vi "Main.vi"(8 "error in (no error)":errorcluster, 11 "Data":T1) -> (0 "error out":errorcluster)   [LabVIEW 2020, in "Queue State Machine Lib.lvlib"]
doc: "Use this template to build a simple state machine design pattern. Each state executes code and determines which state to transition to."
uses:
  Queue State Machine Lib.lvlib
  controls/Data.ctl
  State Machine Data Class/State Machine Data Class.lvclass
  controls/State.ctl
  <vilib>/Delacor/Delacor QMH/Libraries/Message Queue_class/Delacor_lib_QMH_Message Queue.lvclass/Delacor_lib_QMH_Message Queue.ctl
  <vilib>/Delacor/Delacor QMH/Libraries/Message Queue_class/Delacor_lib_QMH_Enqueue Message (Single).vi
  <vilib>/Delacor/Delacor QMH/Libraries/Message Queue_class/Delacor_lib_QMH_Message Queue.lvclass
panel:
  in  "Multiple Consumer?":bool
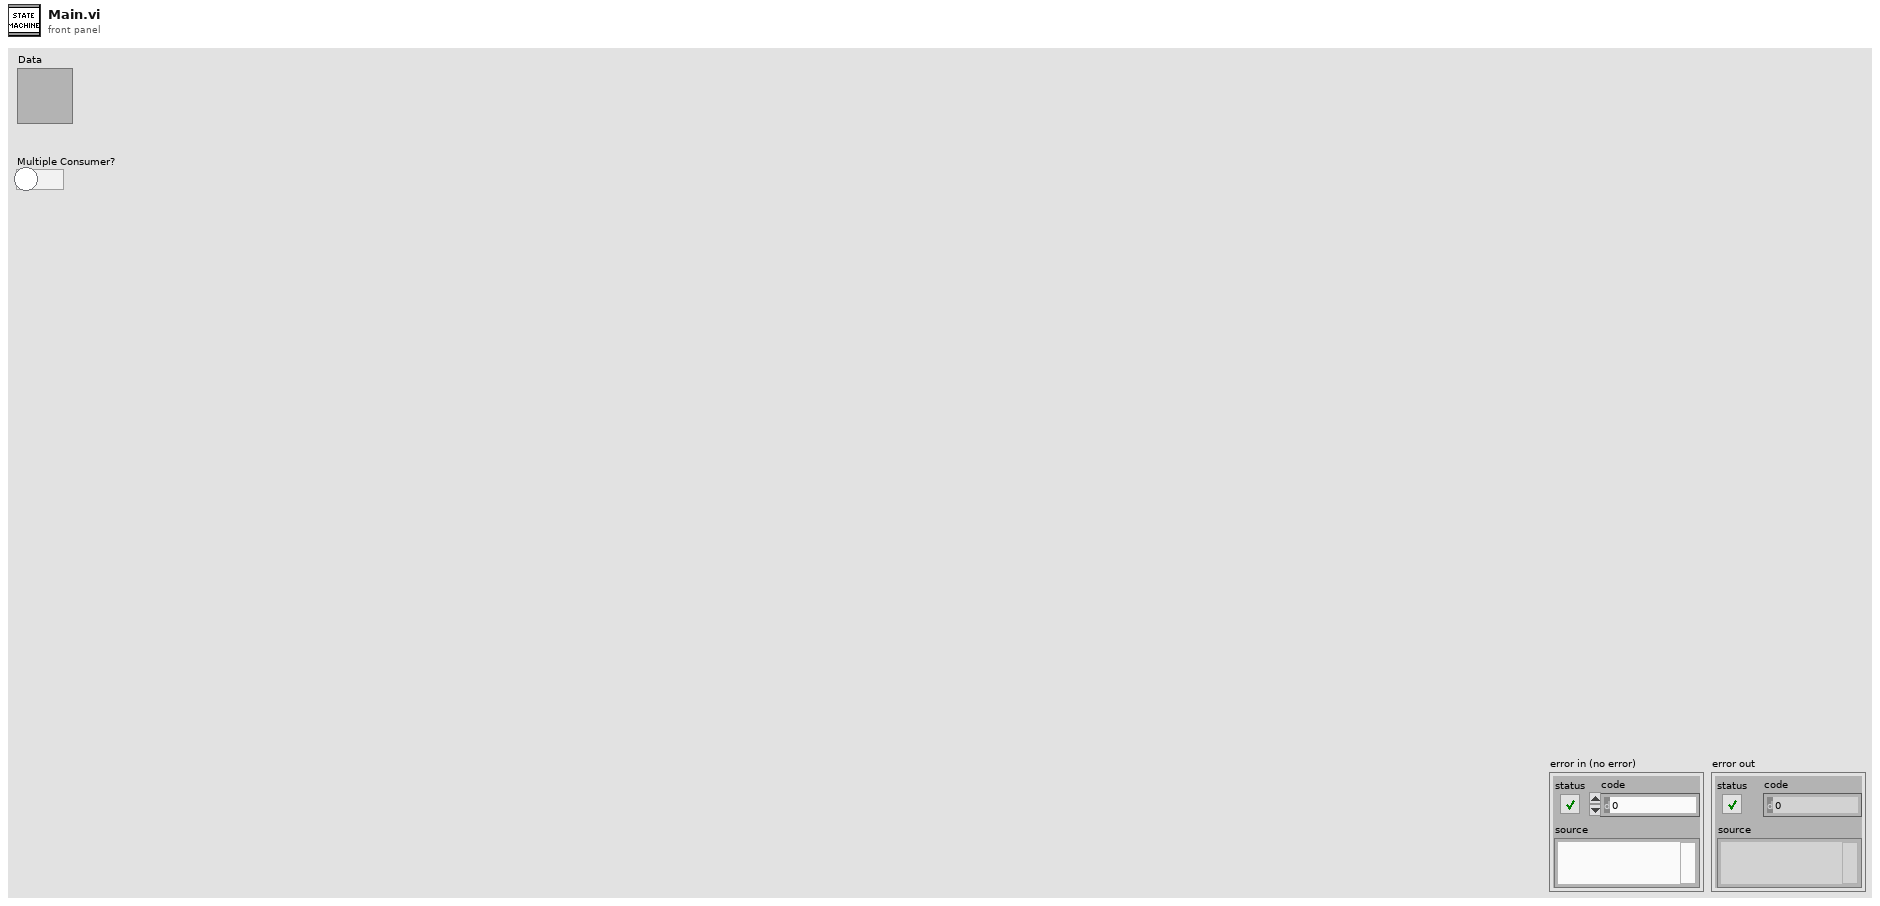
[diagram p1: front panel]
types:
  T1 = typedef "Queue State Machine Lib.lvlib/Data.ctl" = cluster{"Boolean <Replace Me>":bool, "String <Replace Me>":string, "Numeric <Replace Me>":dbl, "tate Machine Data Class.lvclass":refnum<class "State Machine Data Class.lvclass">}
  T2 = typedef "Queue State Machine Lib.lvlib/State.ctl" = enum16{"Initialize", "Wait for Event", "User State 1", "User State 2", "Exit"}
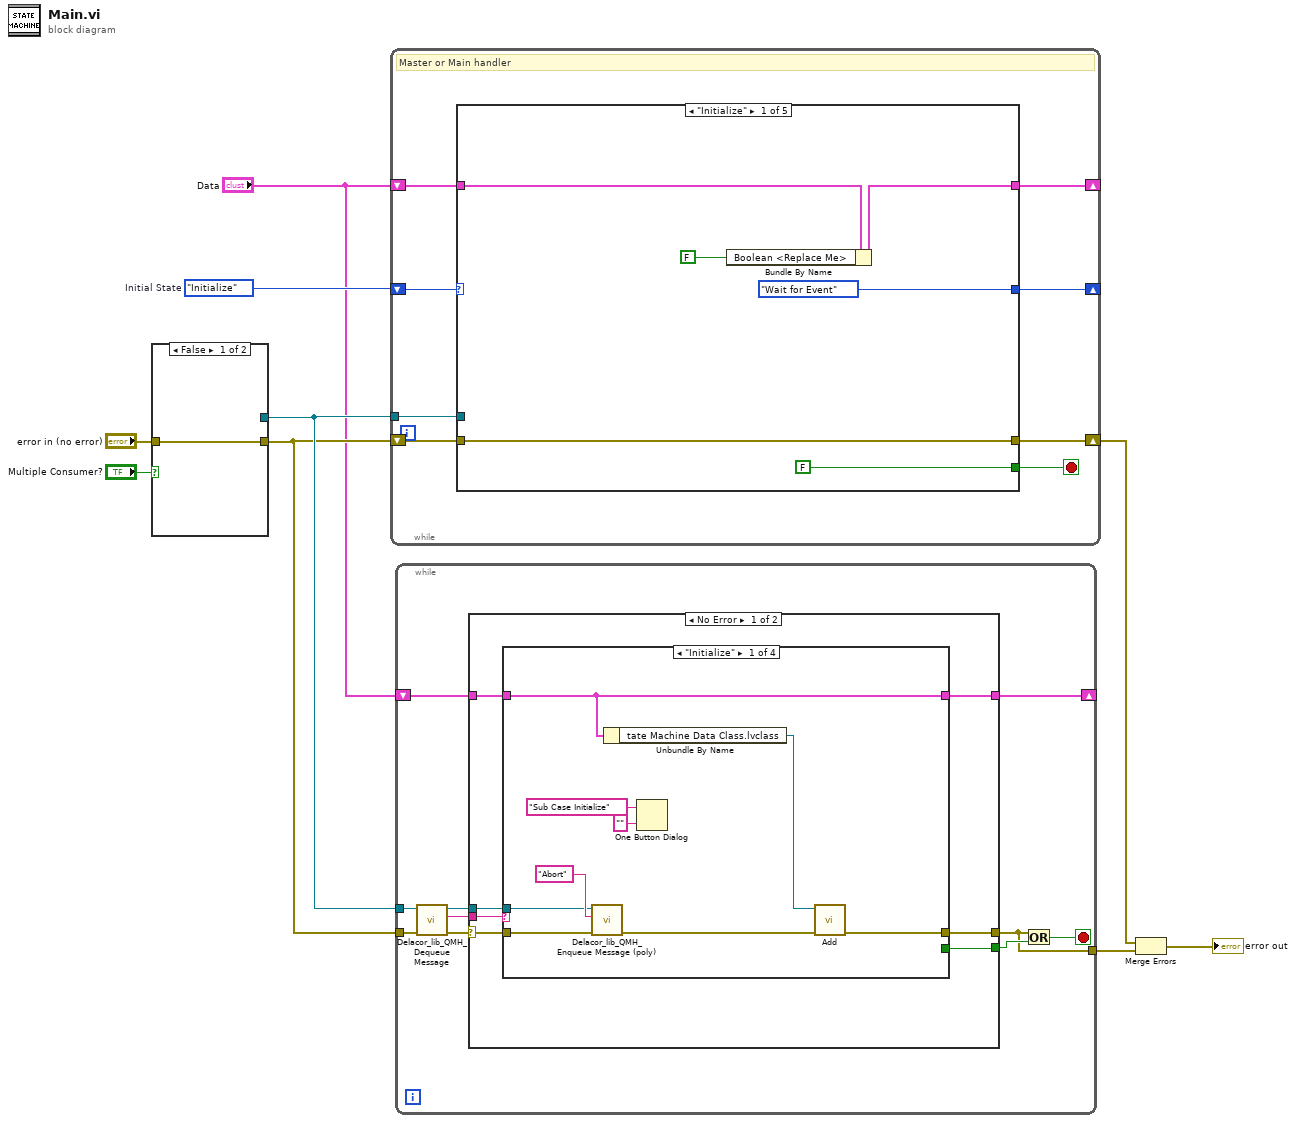
[diagram p0: block diagram]
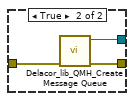
[diagram p2: hidden frame]
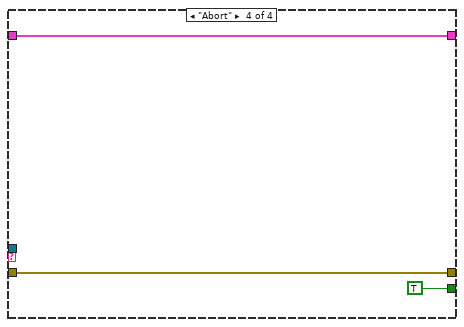
[diagram p5: hidden frame]
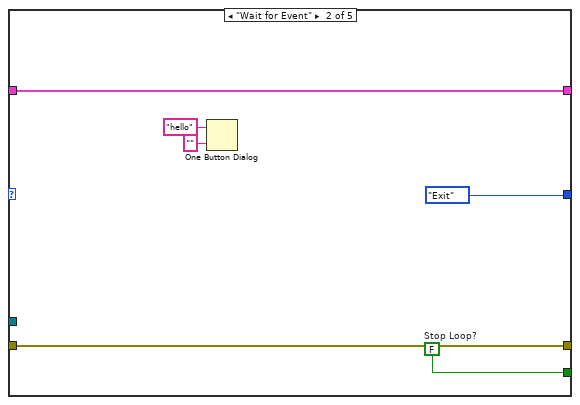
[diagram p7: hidden frame]
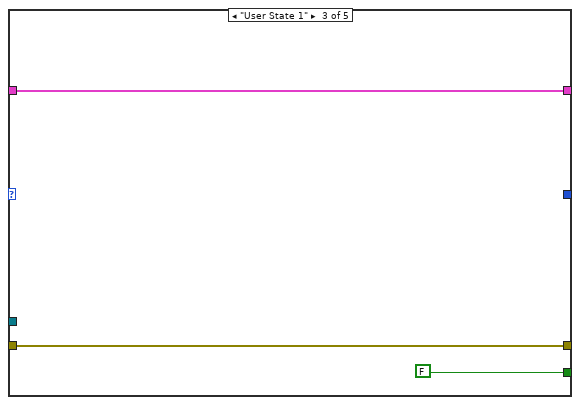
[diagram p8: hidden frame]
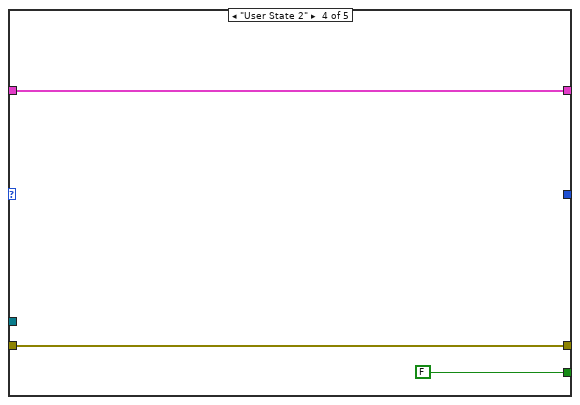
[diagram p9: hidden frame]
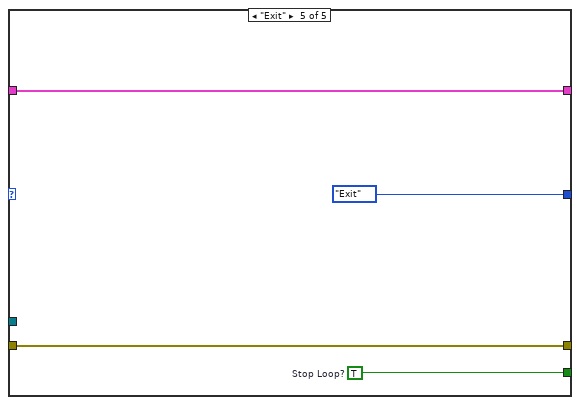
[diagram p10: hidden frame]
diagram:
  w9 = State."Initialize"  # Initial State
  n1 = case shown="False" "Multiple Consumer?" {
    tunnel: "error in (no error)" -> [w10 w13]
    tunnel: [w10 w11] -> w5
    tunnel: [_ w12] -> w6
    frame False {
    }
    frame True {
      n2 = call <vilib>:"Delacor_lib_QMH_Create Message Queue.vi"("error in"=w13) -> ("error out"=w11:errorcluster, "Message Queue"=w12:refnum<class "Delacor_lib_QMH_Message Queue.lvclass">)  [unwired: 9 in]
    }
  }
  n3 = while {
    shift-right: [w20] -> _
    shift-left: w9 -> [w21]
    shift-right: [w18] -> _
    shift-left: "Data" -> [w19]
    shift-right: [w16] -> w2
    shift-left: w5 -> [w17]
    tunnel: w6 -> [w14]
    stop <- w15 stop-if-true
    # "Master or Main handler"
    n4 = case shown="\"Initialize\"" w21 {
      tunnel: [State."Wait for Event" ("Next State") State."Exit" ("(Value Not Used)") _ _ State."Exit" ("(Value Not Used)")] -> w20
      tunnel: [FALSE ("Stop Loop?") w33 FALSE ("Stop Loop?") FALSE ("Stop Loop?") w41] -> w15
      tunnel: w19 -> [w25 w32 w35 w38 w42]
      tunnel: [w24 w32 w35 w38 w42] -> w18
      tunnel: w17 -> [w22 w31 w34 w37 w40]
      tunnel: [w22 w31 w34 w37 w40] -> w16
      tunnel: w14 -> [_ _ _ _ _]
      frame "Initialize" {
        # "Initialize - Initialize the application."
        n5 = Bundle By Name(cluster=w25, "Boolean <Replace Me>"=FALSE ("Replace_Me_Boolean")) -> (w24:T1)
      }
      frame "Wait for Event" {
        w33 = FALSE  # Stop Loop?
        # "Wait for Event - Use an Event Structure to monitor the user interface for events that run different states of the state machine."
        n6 = One Button Dialog(message="hello", button name ("OK")="") -> ()  [unwired: 1 out]
      }
      frame "User State 1" {
        # "User State 1 - Replace this state with functionality for your own application."
      }
      frame "User State 2" {
        # "User State 2 - Replace this state with functionality for your own application."
      }
      frame "Exit" {
        w41 = TRUE  # Stop Loop?
        # "Exit - Exit the application."
      }
    }
  }
  n7 = while {
    tunnel: w6 -> [w52]
    tunnel: w5 -> [w53]
    shift-right: [w45] -> _
    shift-left: "Data" -> [w46]
    tunnel: [w44] -> w3
    stop <- w48 stop-if-true
    n8 = call-dynamic "Delacor_lib_QMH_Dequeue Message.vi"("error in"=w53, "Message Queue in"=w52) -> ("error out"=w50:errorcluster, "Message"=w51:string, "Message Queue out"=w49:refnum<class "Delacor_lib_QMH_Message Queue.lvclass">)  [unwired: 6 in, 1 out]
    n9 = case shown="No Error" w50 {
      selector: w50 -> [w59 w78]
      tunnel: w51 -> [w60 _]
      tunnel: w49 -> [w58 _]
      tunnel: [w56 w78] -> w44
      tunnel: [w57 _] -> w47
      tunnel: w46 -> [w55 w77]
      tunnel: [w54 w77] -> w45
      frame No Error {
        n10 = case shown="\"Initialize\"" w60 {
          tunnel: w59 -> [w66 w71 w73 w76]
          tunnel: [w61 w71 w73 w76] -> w56
          tunnel: w58 -> [w65 _ _ _]
          tunnel: [_ _ _ TRUE ("Stop Loop?")] -> w57
          tunnel: w55 -> [w64 w70 w72 w74]
          tunnel: [w64 w70 w72 w74] -> w54
          frame "Initialize" {
            n11 = call-poly <vilib>:"Delacor_lib_QMH_Enqueue Message (poly).vi"("error in"=w66, "Message"="Abort" ("button name (\"OK\")"), "Message Queue in"=w65) -> ("error out"=w62:errorcluster)  [unwired: 7 in, 1 out]
            n12 = Unbundle By Name(w64) -> ("tate Machine Data Class.lvclass"=w63:refnum<class "State Machine Data Class.lvclass">)
            n13 = One Button Dialog(message="Sub Case Initialize", button name ("OK")="") -> ()  [unwired: 1 out]
            n14 = call-dynamic "Add.vi"("error in (no error)"=w62, "State Machine Data Class in"=w63) -> ("error out"=w61:errorcluster)  [unwired: 8 in, 1 out]
          }
          frame "False", Default {
          }
          frame "True" {
          }
          frame "Abort" {
          }
        }
      }
      frame Error {
      }
    }
    n15 = Or(x=w44, y=w47) -> (x .or. y?=w48:bool)
  }
  n16 = Merge Errors(w2, w3) -> (→"error out":errorcluster)
